vi "Rocket.vi"() -> ()   [LabVIEW 2014]
uses:
  <vilib>/ptbypt/NI_PtbyPt.lvlib
panel:
  out "Output Cluster":T1 {"X Latitude" format="%#.0f"}
  in  "Input Cluster":T2={"Max Speed"=5.0, "Target Offset"=0.0, "Launch"=FALSE, "stop"=FALSE} {"Target Offset" scale=-100.0..100.0; "Max Speed" scale=0.0..5.0}
  out "Rocket":picture
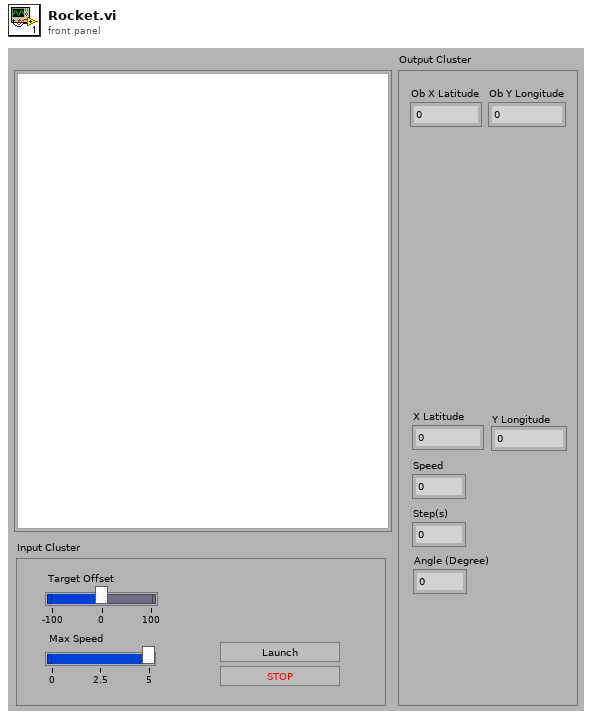
[diagram p1: front panel]
types:
  T1 = cluster{"X Latitude":dbl, "Y Longitude":dbl, "Speed":dbl, "Ob X Latitude":dbl, "Ob Y Longitude":dbl, "Step(s)":dbl, "Angle (Degree)":dbl}
  T2 = cluster{"Max Speed":dbl, "Target Offset":dbl, "Launch":bool, "stop":bool}
  T3 = typedef "imagedata.ctl" = cluster{"image type":i32, "image depth":i32, "image":u8[], "mask":u8[], "colors":u32[], "Rectangle":cluster{"left":i16, "top":i16, "right":i16, "bottom":i16}}
  T4 = cluster{"magnitude":dbl, dbl, "Max Speed":dbl, "magnitude":dbl, dbl, dbl, dbl}
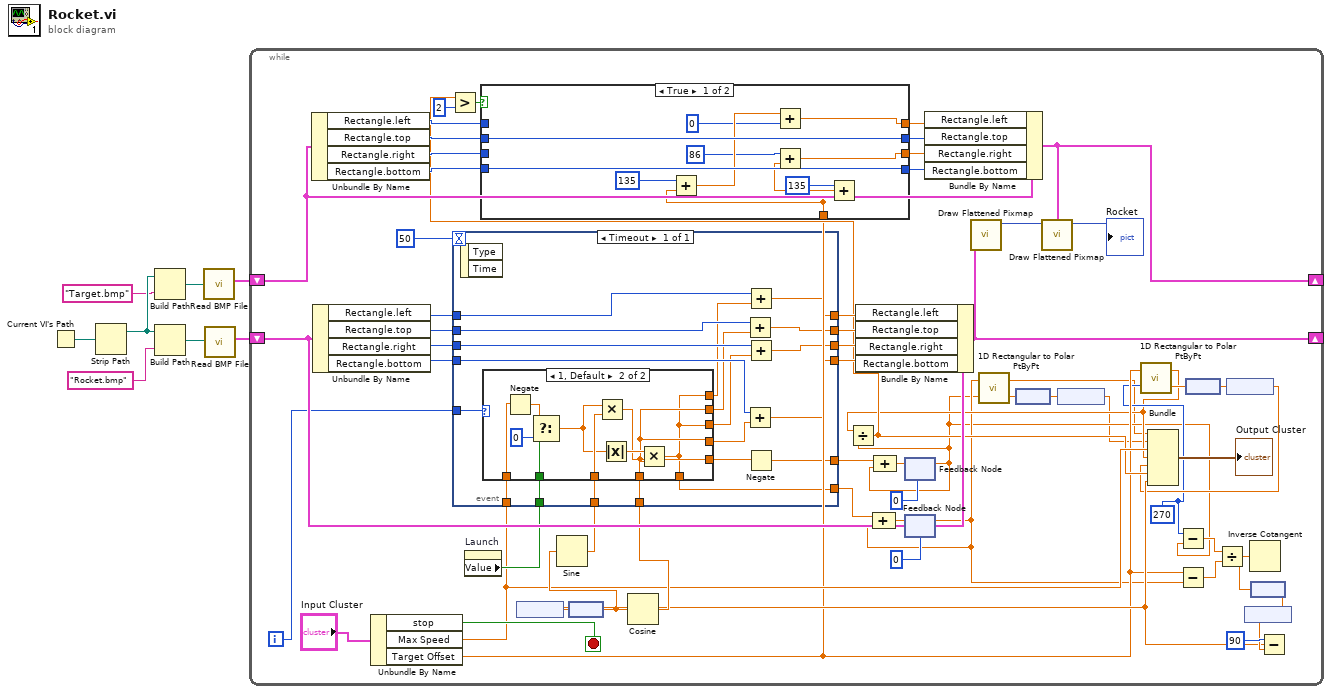
[diagram p0: block diagram]
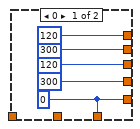
[diagram p3: hidden frame]
diagram:
  n1 = Current VI's Path() -> (path=w8:path)
  n2 = Strip Path(path=w8) -> (stripped path=w6:path)  [unwired: 1 out]
  n3 = Build Path(base path=w6, name or relative path="Target.bmp") -> (appended path=w4:path)
  n4 = Build Path(base path=w6, name or relative path="Rocket.bmp") -> (appended path=w3:path)
  n5 = call <vilib>:"Read BMP File.vi"("path to BMP file"=w4) -> ("image data"=w1:T3)  [unwired: 8 in, 2 out]
  n6 = call <vilib>:"Read BMP File.vi"("path to BMP file"=w3) -> ("image data"=w2:T3)  [unwired: 8 in, 2 out]
  n7 = while {
    shift-right: [w61] -> _
    shift-left: w2 -> [w62]
    shift-right: [w48] -> _
    shift-left: w1 -> [w49]
    i -> [w36]
    stop <- w46 stop-if-true
    w16 = 270
    n8 = Unbundle By Name(w49) -> ("Rectangle.left"=w57:i16, "Rectangle.top"=w56:i16, "Rectangle.right"=w55:i16, "Rectangle.bottom"=w54:i16)
    n9 = Unbundle By Name(w62) -> ("Rectangle.left"=w65:i16, "Rectangle.top"=w70:i16, "Rectangle.right"=w64:i16, "Rectangle.bottom"=w69:i16)
    n10 = Unbundle By Name("Input Cluster") -> ("stop"=w46:bool, "Max Speed"=w32:dbl, "Target Offset"=w20:dbl)
    n11 = property on="Launch" class="Bool (strict)"() -> ("Value"=w35:bool)  [unwired: 2 in, 2 out]
    n12 = feedback #1(0) -> (w11:dbl)
    n13 = feedback #2(0) -> (w12:dbl)
    n14 = call <vilib>:"1D Rectangular to Polar PtByPt.vi"("y"=w11, "x"=w12) -> ("phase"=w14:dbl, "magnitude"=w10:dbl)
    n15 = node(w14) -> (w13:dbl[unit])
    n16 = node ("Convert Unit")(w13) -> (w9:dbl)
    n17 = call <vilib>:"1D Rectangular to Polar PtByPt.vi"("y"=w16, "x"=w20) -> ("phase"=w19:dbl, "magnitude"=w15:dbl)
    n18 = Divide(x=w15, y=w11) -> (x/y=w30:dbl)
    n19 = Greater?(x=w30, y=2) -> (0:w31:bool)
    n20 = case shown="True" w31 {
      tunnel: w57 -> [_ w85]
      tunnel: w56 -> [w81 w84]
      tunnel: w55 -> [_ w83]
      tunnel: w54 -> [w80 w82]
      tunnel: [w79 w85] -> w53
      tunnel: [w81 w84] -> w52
      tunnel: [w78 w83] -> w51
      tunnel: [w80 w82] -> w50
      tunnel: w20 -> [w77 _]
      frame True {
        n21 = Add(x=135, y=w77) -> (x+y=w75:dbl)
        n22 = Add(x=w75, y=0) -> (x+y=w79:dbl)
        n23 = Add(x=135, y=w77) -> (x+y=w73:dbl)
        n24 = Add(x=86, y=w73) -> (x+y=w78:dbl)
      }
      frame False {
      }
    }
    n25 = Bundle By Name(cluster=w49, "Rectangle.left"=w53, "Rectangle.top"=w52, "Rectangle.right"=w51, "Rectangle.bottom"=w50) -> (w48:T3)
    n26 = Subtract(x=w16, y=w11) -> (x-y=w28:dbl)
    n27 = Subtract(x=w20, y=w12) -> (x-y=w27:dbl)
    n28 = node(w19) -> (w18:dbl[unit])
    n29 = Divide(x=w28, y=w27) -> (x/y=w26:dbl)
    n30 = node ("Convert Unit")(w18) -> (w17:dbl)
    n31 = Inverse Cotangent(1:w26) -> (0:w25:dbl)
    n32 = node(w25) -> (w24:dbl[unit])
    n33 = node ("Convert Unit")(w24) -> (w22:dbl)
    n34 = Subtract(x=90, y=w22) -> (x-y=w21:dbl)
    n35 = node ("Convert Unit")(w21) -> (w47:dbl[unit])
    n36 = node(w47) -> (w41:dbl)
    n37 = Sine(x=w41) -> (sin(x)=w42:dbl)
    n38 = Cosine(x=w41) -> (cos(x)=w40:dbl)
    n39 = event shown="[0] Timeout" {
      selector: _ -> [_]
      dyn-events: _ -> [_]
      timeout: 50 -> [_]
      tunnel: w65 -> [w95]
      tunnel: w70 -> [w97]
      tunnel: w64 -> [w99]
      tunnel: w69 -> [w103]
      tunnel: [w93] -> w63
      tunnel: [w96] -> w68
      tunnel: [w100] -> w67
      tunnel: [w102] -> w66
      tunnel: w32 -> [w89]
      tunnel: w36 -> [w105]
      tunnel: w35 -> [w92]
      tunnel: w42 -> [w91]
      tunnel: w40 -> [w90]
      tunnel: [w88] -> w43
      tunnel: [w86] -> w39
      event Timeout {
        n40 = event-data() -> ()  [unwired: 1 in, 2 out]
        n41 = case shown="1, Default" w105 {
          tunnel: [120 w111] -> w94
          tunnel: [300 w112] -> w98
          tunnel: [120 w111] -> w101
          tunnel: [300 w112] -> w104
          tunnel: w92 -> [_ w119]
          tunnel: w91 -> [_ w118]
          tunnel: w90 -> [_ w117]
          tunnel: w89 -> [_ w114]
          tunnel: [w106 w112] -> w87
          tunnel: [w106 w111] -> w88
          frame 0 {
            w106 = 0
          }
          frame 1, Default {
            n42 = Negate(x=w114) -> (-x=w113:dbl)
            n43 = Select(t=w113, s=w119, f=0) -> (s? t:f=w116:dbl)
            n44 = Multiply(x=w116, y=w118) -> (x*y=w112:dbl)
            n45 = Absolute Value(x=w116) -> (abs(x)=w115:dbl)
            n46 = Multiply(x=w115, y=w117) -> (x*y=w111:dbl)
          }
        }
        n47 = Add(x=w97, y=w98) -> (x+y=w96:dbl)
        n48 = Add(x=w103, y=w104) -> (x+y=w102:dbl)
        n49 = Add(x=w95, y=w94) -> (x+y=w93:dbl)
        n50 = Add(x=w99, y=w101) -> (x+y=w100:dbl)
        n51 = Negate(x=w87) -> (-x=w86:dbl)
      }
    }
    n52 = Bundle By Name(cluster=w62, "Rectangle.left"=w63, "Rectangle.top"=w68, "Rectangle.right"=w67, "Rectangle.bottom"=w66) -> (w61:T3)
    n53 = Compound Arithmetic op=ADD(w43, w12) -> (w44:dbl)
    n54 = Compound Arithmetic op=ADD(w39, w11) -> (w45:dbl)
    n55 = feedback-in #1(w45) -> ()
    n56 = feedback-in #2(w44) -> ()
    n57 = call <vilib>:"Draw Flattened Pixmap.vi"("image data"=w61) -> ("new picture"=w59:picture)  [unwired: 8 in]
    n58 = call <vilib>:"Draw Flattened Pixmap.vi"("image data"=w48, "picture"=w59) -> ("new picture"=→"Rocket":picture)  [unwired: 7 in]
    n59 = Bundle("magnitude"=w10, w9, "Max Speed"=w32, "magnitude"=w15, w17, w30, w21) -> (→"Output Cluster":T4)  [unwired: 1 in]
  }
